vi "indexed_sort.vi"(2 "n":i32, 3 "A":sgl[](array[numeric])=[0.0, 0.0, 0.0, 0.0, 0.0, 0.0, 0.0, 0.0, 0.0, 0.0, 0.0, 0.0, 0.0, 0.0, 0.0, 0.0, 0.0, 0.0, 0.0, 0.0]) -> (0 "Index":i32[](array[numeric]), 1 "Sorted A":sgl[](array[numeric]))   [LabVIEW 2020]
uses:
  <vilib>/rvi/Emulation/niFpgaGetClockAttributes.vi
  <vilib>/rvi/Emulation/niFpgaSctlEmulationGetInTimedLoop.vi
  <vilib>/rvi/Emulation/niFpgaEmulationReportErrorSimple.vi
  <vilib>/rvi/Emulation/niFpgaCriticalErrorInLSC.vi
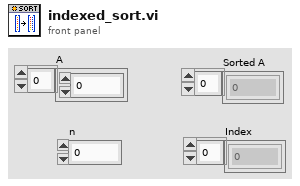
[diagram p1: front panel]
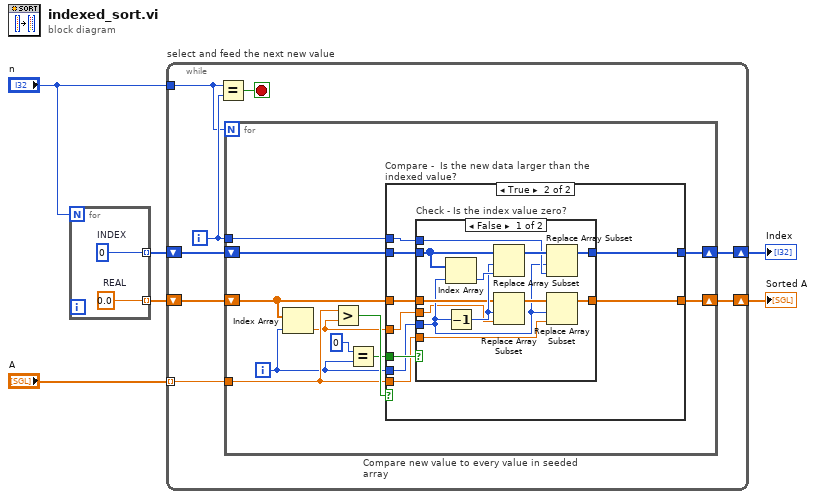
[diagram p0: block diagram]
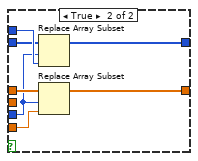
[diagram p3: hidden frame]
diagram:
  n1 = for {
    N: "n" -> [_]
    tunnel: [w8] -> w3 mode=indexing
    tunnel: [w7] -> w4 mode=indexing
    w7 = 0  # INDEX
    w8 = sgl 0.0  # REAL
  }
  n2 = while "select and feed the next new value" {
    shift-right: [w15] -> w5
    shift-left: w3 -> [w16]
    shift-right: [w14] -> w6
    shift-left: w4 -> [w13]
    tunnel: "n" -> [w9]
    tunnel: "A" -> [w10] mode=indexing
    i -> [w12]
    stop <- w11 stop-if-true
    n3 = Equal?(x=w9, y=w12) -> (x = y?=w11:bool)
    n4 = for "Compare new value to every value in seeded array" {
      N: w9 -> [_]
      tunnel: w10 -> [w25]
      shift-right: [w24] -> w15
      shift-left: w16 -> [w26]
      tunnel: w12 -> [w22]
      shift-right: [w20] -> w14
      shift-left: w13 -> [w21]
      i -> [w23]
      n5 = Index Array(array=w26, index=w23) -> (element=w17:sgl)
      n6 = Greater?(x=w25, y=w17) -> (0:w27:bool)
      n7 = Equal?(x=0, y=w23) -> (x = y?=w18:bool)
      n8 = case "Compare -  Is the new data larger than the indexed value?" shown="True" w27 {
        tunnel: w26 -> [w29 w37]
        tunnel: w18 -> [_ w38]
        tunnel: w25 -> [_ w36]
        tunnel: w23 -> [_ w35]
        tunnel: [w29 w34] -> w24
        tunnel: w22 -> [_ w33]
        tunnel: w21 -> [w28 w32]
        tunnel: [w28 w31] -> w20
        tunnel: w17 -> [_ w30]
        frame False {
        }
        frame True {
          n9 = case "Check - Is the index value zero?" shown="False" w38 {
            tunnel: w37 -> [w41 w57]
            tunnel: w36 -> [w49 w56]
            tunnel: w35 -> [w40 w51]
            tunnel: [w48 w55] -> w34
            tunnel: w33 -> [w43 w54]
            tunnel: w32 -> [w45 w53]
            tunnel: [w44 w52] -> w31
            tunnel: w30 -> [w39 _]
            frame False {
              n10 = Index Array(array=w45, index=w40) -> (element=w47:i32)
              n11 = Decrement(x=w40) -> (x-1=w42:i32)
              n12 = Replace Array Subset(array=w45, new element=w47, index=w42) -> (w46:i32[])
              n13 = Replace Array Subset(array=w41, new element=w39, index=w42) -> (w50:sgl[])
              n14 = Replace Array Subset(array=w46, new element=w43, index=w40) -> (w44:i32[])
              n15 = Replace Array Subset(array=w50, new element=w49, index=w40) -> (w48:sgl[])
            }
            frame True {
              n16 = Replace Array Subset(array=w53, new element=w54, index=w51) -> (w52:i32[])
              n17 = Replace Array Subset(array=w57, new element=w56, index=w51) -> (w55:sgl[])
            }
          }
        }
      }
    }
  }
  "Index" <- w6
  "Sorted A" <- w5
